vi "Lab Panel V4.91.vi"() -> ()   [LabVIEW 2013] (continued)
              n208 = local read "SIG LAB02-1"() -> (w244:T2)
              n209 = local read "SIG LAB02-2"() -> (w243:T2)
              n210 = local read "TEMP LA02"() -> (w248:T9)
              n211 = Bundle By Name(cluster=w248, "TL-1"=w240, "TN-1"=w239, "TL-2"=w238, "TN-2"=w237, "TL -1COUNT"=w245, "TN-1 COUNT"=w245, "TL-2 COUNT"=w245, "TN-2 COUNT"=w245) -> (w246:T9)
              n212 = Bundle(cluster=w243, "Tmp Live"=w238, "Tmp Neut"=w237) -> (w241:T2)  [unwired: 3 in]
              n213 = Bundle(cluster=w244, "Tmp Live"=w240, "Tmp Neut"=w239) -> (w242:T2)  [unwired: 3 in]
              n214 = local write "TEMP LA02"(w246) -> ()
              n215 = local write "SIG LAB02-1"(w242) -> ()
              n216 = local write "SIG LAB02-2"(w241) -> ()
            }
            frame #4 {
              w257 = 0
              n217 = local read "LAB03 TEMP"() -> (w259:T12)
              n218 = Unbundle By Name(w259) -> ("T1 Live"=w252:dbl, "T1 Neut"=w251:dbl, "T2 Live"=w250:dbl, "T2 Neut"=w249:dbl)  [unwired: 2 out]
              n219 = local read "SIG LAB03-1"() -> (w256:T2)
              n220 = local read "SIG LAB03-2"() -> (w255:T2)
              n221 = local read "TEMP LA03"() -> (w260:T9)
              n222 = Bundle By Name(cluster=w260, "TL-1"=w252, "TN-1"=w251, "TL-2"=w250, "TN-2"=w249, "TL -1COUNT"=w257, "TN-1 COUNT"=w257, "TL-2 COUNT"=w257, "TN-2 COUNT"=w257) -> (w258:T9)
              n223 = Bundle(cluster=w255, "Tmp Live"=w250, "Tmp Neut"=w249) -> (w253:T2)  [unwired: 3 in]
              n224 = Bundle(cluster=w256, "Tmp Live"=w252, "Tmp Neut"=w251) -> (w254:T2)  [unwired: 3 in]
              n225 = local write "TEMP LA03"(w258) -> ()
              n226 = local write "SIG LAB03-2"(w253) -> ()
              n227 = local write "SIG LAB03-1"(w254) -> ()
            }
            frame #5 {
              w269 = 0
              n228 = local read "LAB04 TEMP"() -> (w271:T12)
              n229 = Unbundle By Name(w271) -> ("T1 Live"=w264:dbl, "T1 Neut"=w263:dbl, "T2 Live"=w262:dbl, "T2 Neut"=w261:dbl)  [unwired: 2 out]
              n230 = local read "SIG LAB04-2"() -> (w267:T2)
              n231 = local read "SIG LAB04-1"() -> (w268:T2)
              n232 = local read "TEMP LA04"() -> (w272:T9)
              n233 = Bundle By Name(cluster=w272, "TL-1"=w264, "TN-1"=w263, "TL-2"=w262, "TN-2"=w261, "TL -1COUNT"=w269, "TN-1 COUNT"=w269, "TL-2 COUNT"=w269, "TN-2 COUNT"=w269) -> (w270:T9)
              n234 = Bundle(cluster=w267, "Tmp Live"=w262, "Tmp Neut"=w261) -> (w265:T2)  [unwired: 3 in]
              n235 = Bundle(cluster=w268, "Tmp Live"=w264, "Tmp Neut"=w263) -> (w266:T2)  [unwired: 3 in]
              n236 = local write "SIG LAB04-2"(w265) -> ()
              n237 = local write "TEMP LA04"(w270) -> ()
              n238 = local write "SIG LAB04-1"(w266) -> ()
            }
            frame #6 {
              w281 = 0
              n239 = local read "LAB05 TEMP"() -> (w283:T12)
              n240 = Unbundle By Name(w283) -> ("T1 Live"=w276:dbl, "T1 Neut"=w275:dbl, "T2 Live"=w274:dbl, "T2 Neut"=w273:dbl)  [unwired: 2 out]
              n241 = local read "SIG LAB05-2"() -> (w279:T2)
              n242 = local read "SIG LAB05-1"() -> (w280:T2)
              n243 = local read "TEMP LA05"() -> (w284:T9)
              n244 = Bundle By Name(cluster=w284, "TL-1"=w276, "TN-1"=w275, "TL-2"=w274, "TN-2"=w273, "TL -1COUNT"=w281, "TN-1 COUNT"=w281, "TL-2 COUNT"=w281, "TN-2 COUNT"=w281) -> (w282:T9)
              n245 = Bundle(cluster=w279, "Tmp Live"=w274, "Tmp Neut"=w273) -> (w277:T2)  [unwired: 3 in]
              n246 = Bundle(cluster=w280, "Tmp Live"=w276, "Tmp Neut"=w275) -> (w278:T2)  [unwired: 3 in]
              n247 = local write "SIG LAB05-2"(w277) -> ()
              n248 = local write "SIG LAB05-1"(w278) -> ()
              n249 = local write "TEMP LA05"(w282) -> ()
            }
          }
        }
        frame #8 {
          # "enable front panel, all settings done"
          n250 = property on="Tab Control 2" class="TabCtl (strict)"("DisabledEnum"=T16."Enabled" ("Disabled")) -> ()  [unwired: 2 in, 2 out]
          n251 = property on="Tab Control 2" class="TabCtl (strict)"("Value"=0) -> ()  [unwired: 2 in, 2 out]
        }
        frame #9 {
          n252 = property on="Tab Control 2" class="TabCtl (strict)"("Value"=0) -> ()  [unwired: 2 in, 2 out]
        }
      }
    }
    frame #2 {
      n253 = node-c288("loop  delay(mS)") -> (w290:T17)  [unwired: 3 in]
      n254 = timed-loop {
        timing: w290 -> [_]
        timing-out: [_] -> w289
        i -> [w312]
        stop <- "stop" stop-if-true
        n255 = node-c288() -> ()  [unwired: 1 in, 1 out]
        n256 = global write "Global display 1.vi" "stop disp"("stop") -> ()
        n257 = local read "SELECT LAB05-2"() -> (w292:T3)
        n258 = local read "SELECT LAB05-1"() -> (w293:T3)
        n259 = local read "SELECT LAB04-2"() -> (w294:T3)
        n260 = local read "SELECT LAB03-1"() -> (w297:T3)
        n261 = local read "SELECT LAB02-2"() -> (w298:T3)
        n262 = local read "SELECT LAB01-1"() -> (w301:T3)
        n263 = local read "SELECT LAB03-2"() -> (w296:T3)
        n264 = local read "SELECT LAB01-2"() -> (w300:T3)
        n265 = local read "SELECT LAB04-1"() -> (w295:T3)
        n266 = local read "SELECT LAB02-1"() -> (w299:T3)
        n267 = local read "run lab03-2"() -> (w306:bool)
        n268 = local read "run lab04-1"() -> (w305:bool)
        n269 = local read "run lab05-1"() -> (w303:bool)
        n270 = local read "run lab04-2"() -> (w304:bool)
        n271 = local read "run lab05-2"() -> (w302:bool)
        n272 = local read "run lab03-1"() -> (w307:bool)
        n273 = local read "run lab02-2"() -> (w308:bool)
        n274 = local read "run lab02-1"() -> (w309:bool)
        n275 = local read "run lab01-1"() -> (w311:bool)
        n276 = local read "run lab01-2"() -> (w310:bool)
        n277 = stacked-sequence {
          seq-local: [_ w377 _ _ _ _ _ _ _ _ _ _ _ _ _ _ _ _ _ _ _ _ _] -> [_ _ _ _ _ w2478 _ _ _ _ _ _ _ _ _ _ _ _ _ _ _ _ _]
          seq-local: [_ w376 _ _ _ _ _ _ _ _ _ _ _ _ _ _ _ _ _ _ _ _ _] -> [_ _ _ _ _ w2477 _ _ _ _ _ _ _ _ _ _ _ _ _ _ _ _ _]
          seq-local: [_ w363 _ _ _ _ _ _ _ _ _ _ _ _ _ _ _ _ _ _ _ _ _] -> [_ _ _ _ _ w2476 _ _ _ _ _ _ _ _ _ _ _ _ _ _ _ _ _]
          seq-local: [_ w362 _ _ _ _ _ _ _ _ _ _ _ _ _ _ _ _ _ _ _ _ _] -> [_ _ _ _ _ w2475 _ _ _ _ _ _ _ _ _ _ _ _ _ _ _ _ _]
          seq-local: [_ w361 _ _ _ _ _ _ _ _ _ _ _ _ _ _ _ _ _ _ _ _ _] -> [_ _ _ _ _ w2474 _ _ _ _ _ _ _ _ _ _ _ _ _ _ _ _ _]
          seq-local: [_ w360 _ _ _ _ _ _ _ _ _ _ _ _ _ _ _ _ _ _ _ _ _] -> [_ _ _ _ _ w2473 _ _ _ _ _ _ _ _ _ _ _ _ _ _ _ _ _]
          seq-local: [_ w359 _ _ _ _ _ _ _ _ _ _ _ _ _ _ _ _ _ _ _ _ _] -> [_ _ _ _ _ w2472 _ _ _ _ _ _ _ _ _ _ _ _ _ _ _ _ _]
          seq-local: [_ w358 _ _ _ _ _ _ _ _ _ _ _ _ _ _ _ _ _ _ _ _ _] -> [_ _ _ _ _ w2471 _ _ _ _ _ _ _ _ _ _ _ _ _ _ _ _ _]
          seq-local: [_ w357 _ _ _ _ _ _ _ _ _ _ _ _ _ _ _ _ _ _ _ _ _] -> [_ _ _ _ _ w2470 _ _ _ _ _ _ _ _ _ _ _ _ _ _ _ _ _]
          seq-local: [_ w356 _ _ _ _ _ _ _ _ _ _ _ _ _ _ _ _ _ _ _ _ _] -> [_ _ _ _ _ w2469 _ _ _ _ _ _ _ _ _ _ _ _ _ _ _ _ _]
          tunnel: w311 -> [_ _ w393 w641 w2068 w2498 w2813 w3300 _ _ _ _ w3725 _ w4682 _ _ w4969 w5272 w5454 _ _ _]
          tunnel: w310 -> [_ _ w392 w639 w2067 w2497 w2814 w3299 _ _ _ _ w3724 _ w4680 _ _ w4968 w5271 w5452 _ _ _]
          tunnel: w309 -> [_ _ w391 w637 w2066 w2496 w2812 w3298 _ _ _ _ w3723 _ w4678 _ _ w4967 w5270 w5451 _ _ _]
          tunnel: w308 -> [_ _ w390 w635 w2065 w2495 w2811 w3297 _ _ _ _ w3722 _ w4676 _ _ w4966 w5269 w5450 _ _ _]
          tunnel: w307 -> [_ _ w389 w633 w2064 w2494 w2810 w3296 _ _ _ _ w3721 _ w4674 _ _ w4965 w5268 w5449 _ _ _]
          tunnel: w306 -> [_ _ w388 w631 w2063 w2493 w2809 w3295 _ _ _ _ w3720 _ w4672 _ _ w4964 w5267 w5448 _ _ _]
          tunnel: w305 -> [_ _ w387 w629 w2062 w2492 w2808 w3294 _ _ _ _ w3719 _ w4670 _ _ w4963 w5266 w5447 _ _ _]
          tunnel: w304 -> [_ _ w386 w627 w2061 w2491 w2807 w3293 _ _ _ _ w3718 _ w4668 _ _ w4962 w5265 w5446 _ _ _]
          tunnel: w303 -> [_ _ w385 w625 w2060 w2490 w2806 w3292 _ _ _ _ w3717 _ w4666 _ _ w4961 w5264 w5445 _ _ _]
          tunnel: w302 -> [_ _ w384 w623 w2059 w2489 w2805 w3291 _ _ _ _ w3716 _ w4664 _ _ w4960 w5263 w5444 _ _ _]
          tunnel: w301 -> [_ _ _ w640 w2058 w2488 _ _ _ _ _ _ _ _ w4684 _ _ _ _ _ w5792 _ _]
          tunnel: w300 -> [_ _ _ w638 w2057 w2487 _ _ _ _ _ _ _ _ w4679 _ _ _ _ _ w5791 _ _]
          tunnel: w299 -> [_ _ _ w636 w2056 w2486 _ _ _ _ _ _ _ _ w4677 _ _ _ _ _ w5790 _ _]
          tunnel: w298 -> [_ _ _ w634 w2055 w2485 _ _ _ _ _ _ _ _ w4675 _ _ _ _ _ w5789 _ _]
          tunnel: w297 -> [_ _ _ w632 w2054 w2484 _ _ _ _ _ _ _ _ w4673 _ _ _ _ _ w5788 _ _]
          tunnel: w296 -> [_ _ _ w630 w2053 w2483 _ _ _ _ _ _ _ _ w4671 _ _ _ _ _ w5787 _ _]
          tunnel: w295 -> [_ _ _ w628 w2052 w2482 _ _ _ _ _ _ _ _ w4669 _ _ _ _ _ w5786 _ _]
          tunnel: w294 -> [_ _ _ w626 w2051 w2481 _ _ _ _ _ _ _ _ w4667 _ _ _ _ _ w5785 _ _]
          tunnel: w293 -> [_ _ _ w624 w2050 w2480 _ _ _ _ _ _ _ _ w4665 _ _ _ _ _ w5784 _ _]
          tunnel: w292 -> [_ _ _ w622 w2049 w2479 _ _ _ _ _ _ _ _ w4663 _ _ _ _ _ w5783 _ _]
          frame #0 {
            w319 = FALSE
            w324 = 0.5
            # "set up cycle control"
            n278 = local read "jig cycle"() -> (w323:dbl)
            n279 = local read "Amps Fail level"() -> (w317:dbl)
            n280 = Divide(x="JIG ON TIME (S)", y=w324) -> (x/y=→"on loops":dbl)
            n281 = Divide(x="JIG OFF TIME (S)", y=w324) -> (x/y=→"off loops":dbl)
            n282 = global write "Global display 3.vi" "Amps Fail"(w317) -> ()
            n283 = Increment(x=w323) -> (x+1=w322:dbl)
            n284 = local write "TEMP"(w319) -> ()
            n285 = local write "AI"(w319) -> ()
            n286 = local read "Network Directory"() -> (w316:path)
            n287 = local write "jig cycle"(w322) -> ()
            n288 = call "sub vi - check network dir v2.vi"("PATH"=w316) -> ("error"=w315:bool)  [unwired: 10 in]
            n289 = local write "network error"(w315) -> ()
            n290 = global write "Global display 3.vi" "network drive"(w315) -> ()
            n291 = event shown="[1] \"ADMIN\": Value Change" {
              selector: _ -> [_ _]
              dyn-events: _ -> [_ _]
              timeout: 10 -> [_ _]
              event Timeout {
                n292 = event-data() -> ()  [unwired: 1 in, 3 out]
              }
              event "ADMIN": Value Change {
                n293 = event-data() -> ()  [unwired: 1 in, 6 out]
                n294 = stacked-sequence {
                  seq-local: [_ w328 _] -> [_ _ w329]
                  frame #0 {
                    n295 = global write "Global 1.vi" "password"("9949") -> ()
                  }
                  frame #1 {
                    n296 = call "sub vi - password 1.vi"() -> ("RESULT"=w328:bool)  [unwired: 11 in]
                  }
                  frame #2 {
                    w331 = FALSE
                    n297 = property on="Tab Control 2" class="TabCtl (strict)"() -> ("Pages"=w335:refnum<vi>[])  [unwired: 2 in, 2 out]
                    n298 = Select(t=TRUE, s=w329, f=w331) -> (s? t:f=w330:bool)
                    n299 = Index Array(array=w335, index=8) -> (element=w333:refnum<vi>)
                    n300 = property class="Page"(reference=w333, "PageVis"=w330) -> ()  [unwired: 1 in, 2 out]
                    n301 = local write "ADMIN"(w331) -> ()
                  }
                }
              }
            }
          }
          frame #1 {
            w373 = 60.0
            # "convert temperature rise minutes to cycles"
            n302 = local read "SET LAB05-2"() -> (w337:T5)
            n303 = local read "SET LAB05-1"() -> (w339:T5)
            n304 = local read "SET LAB04-2"() -> (w341:T5)
            n305 = local read "SET LAB01-1"() -> (w355:T5)
            n306 = local read "SET LAB01-2"() -> (w353:T5)
            n307 = local read "SET LAB02-2"() -> (w349:T5)
            n308 = local read "SET LAB04-1"() -> (w343:T5)
            n309 = local read "SET LAB03-1"() -> (w347:T5)
            n310 = local read "SET LAB03-2"() -> (w345:T5)
            n311 = local read "SET LAB02-1"() -> (w351:T5)
            n312 = local read "JIG OFF TIME (S)"() -> (w378:dbl)
            n313 = local read "JIG ON TIME (S)"() -> (w379:dbl)
            n314 = Unbundle(w337) -> ("T-RISE mins"=w336:dbl)  [unwired: 4 out]
            n315 = Unbundle(w339) -> ("T-RISE mins"=w338:dbl)  [unwired: 4 out]
            n316 = Unbundle(w355) -> ("T-RISE mins"=w354:dbl)  [unwired: 4 out]
            n317 = Unbundle(w341) -> ("T-RISE mins"=w340:dbl)  [unwired: 4 out]
            n318 = Unbundle(w353) -> ("T-RISE mins"=w352:dbl)  [unwired: 4 out]
            n319 = Unbundle(w351) -> ("T-RISE mins"=w350:dbl)  [unwired: 4 out]
            n320 = Unbundle(w343) -> ("T-RISE mins"=w342:dbl)  [unwired: 4 out]
            n321 = Unbundle(w349) -> ("T-RISE mins"=w348:dbl)  [unwired: 4 out]
            n322 = Unbundle(w345) -> ("T-RISE mins"=w344:dbl)  [unwired: 4 out]
            n323 = Unbundle(w347) -> ("T-RISE mins"=w346:dbl)  [unwired: 4 out]
            n324 = Add(x=w379, y=w378) -> (x+y=w372:dbl)
            n325 = Multiply(x=w373, y=w344) -> (x*y=w368:dbl)
            n326 = Multiply(x=w373, y=w342) -> (x*y=w367:dbl)
            n327 = Multiply(x=w373, y=w340) -> (x*y=w366:dbl)
            n328 = Multiply(x=w373, y=w338) -> (x*y=w365:dbl)
            n329 = Multiply(x=w373, y=w336) -> (x*y=w364:dbl)
            n330 = Multiply(x=w373, y=w352) -> (x*y=w374:dbl)
            n331 = Multiply(x=w373, y=w346) -> (x*y=w369:dbl)
            n332 = Multiply(x=w373, y=w354) -> (x*y=w375:dbl)
            n333 = Multiply(x=w373, y=w350) -> (x*y=w371:dbl)
            n334 = Multiply(x=w373, y=w348) -> (x*y=w370:dbl)
            n335 = Divide(x=w365, y=w372) -> (x/y=w357:dbl)
            n336 = Divide(x=w366, y=w372) -> (x/y=w358:dbl)
            n337 = Divide(x=w367, y=w372) -> (x/y=w359:dbl)
            n338 = Divide(x=w364, y=w372) -> (x/y=w356:dbl)
            n339 = Divide(x=w369, y=w372) -> (x/y=w361:dbl)
            n340 = Divide(x=w375, y=w372) -> (x/y=w377:dbl)
            n341 = Divide(x=w374, y=w372) -> (x/y=w376:dbl)
            n342 = Divide(x=w371, y=w372) -> (x/y=w363:dbl)
            n343 = Divide(x=w370, y=w372) -> (x/y=w362:dbl)
            n344 = Divide(x=w368, y=w372) -> (x/y=w360:dbl)
          }
          frame #2 {
            # "control cycle loops"
            n345 = local read "JIG OFF TIME (S)"() -> (w382:dbl)
            n346 = local read "JIG ON TIME (S)"() -> (w381:dbl)
            n347 = local read "jig cycle"() -> (w395:dbl)
            n348 = local read "on loops"() -> (w397:dbl)
            n349 = local read "off loops"() -> (w396:dbl)
            n350 = Add(x=w382, y=w381) -> (x+y=w380:dbl)
            n351 = Add(x=w397, y=w396) -> (x+y=w383:dbl)
            n352 = Greater Or Equal?(x=w395, y=w383) -> (x >= y?=w394:bool)
            n353 = case shown="True" w394 {
              tunnel: w393 -> [_ w431]
              tunnel: w392 -> [_ w430]
              tunnel: w391 -> [_ w429]
              tunnel: w390 -> [_ w428]
              tunnel: w389 -> [_ w427]
              tunnel: w388 -> [_ w426]
              tunnel: w387 -> [_ w425]
              tunnel: w386 -> [_ w424]
              tunnel: w385 -> [_ w423]
              tunnel: w384 -> [_ w422]
              tunnel: w380 -> [_ w421]
              frame False {
              }
              frame True {
                # "increment cycle value and convert cycles to minutes for temp rise"
                n354 = stacked-sequence {
                  frame #0 {
                    n355 = local read "Panel #"() -> (w434:dbl)
                    n356 = Increment(x=w434) -> (x+1=w433:dbl)
                    n357 = local write "Panel #"(w433) -> ()
                  }
                  frame #1 {
                    n358 = local read "Panel #"() -> (w435:dbl)
                    n359 = Greater?(x=w435, y=5) -> (0:w437:bool)
                    n360 = case shown="True" w437 {
                      frame False {
                      }
                      frame True {
                        n361 = local write "Panel #"(1) -> ()
                      }
                    }
                  }
                }
                n362 = local read "JIG RELAY CYCLES"() -> (w420:T8)
                n363 = local read "Panel #"() -> (→"Tmp Upd":dbl)
                n364 = Unbundle By Name(w420) -> ("LAB01-1"=w418:dbl, "LAB01-2"=w416:dbl, "LAB02-1"=w414:dbl, "LAB02-2"=w412:dbl, "LAB03-1"=w410:dbl, "LAB03-2"=w408:dbl, "LAB04-1"=w406:dbl, "LAB04-2"=w404:dbl, "LAB05-1"=w402:dbl, "LAB05-2"=w400:dbl)
                n365 = stacked-sequence {
                  tunnel: w431 -> [w449 _ _ _ _ _ _ _ _ _]
                  tunnel: w430 -> [_ w466 _ _ _ _ _ _ _ _]
                  tunnel: w429 -> [_ _ w483 _ _ _ _ _ _ _]
                  tunnel: w428 -> [_ _ _ w500 _ _ _ _ _ _]
                  tunnel: w427 -> [_ _ _ _ w517 _ _ _ _ _]
                  tunnel: w426 -> [_ _ _ _ _ w534 _ _ _ _]
                  tunnel: w425 -> [_ _ _ _ _ _ w551 _ _ _]
                  tunnel: w424 -> [_ _ _ _ _ _ _ w568 _ _]
                  tunnel: w423 -> [_ _ _ _ _ _ _ _ w585 _]
                  tunnel: w422 -> [_ _ _ _ _ _ _ _ _ w602]
                  tunnel: w421 -> [w446 w463 w480 w497 w514 w531 w548 w565 w582 w599]
                  tunnel: w418 -> [w440 _ _ _ _ _ _ _ _ _]
                  tunnel: [w439 _ _ _ _ _ _ _ _ _] -> w417
                  tunnel: w416 -> [_ w457 _ _ _ _ _ _ _ _]
                  tunnel: [_ w456 _ _ _ _ _ _ _ _] -> w415
                  tunnel: w414 -> [_ _ w474 _ _ _ _ _ _ _]
                  tunnel: [_ _ w473 _ _ _ _ _ _ _] -> w413
                  tunnel: w412 -> [_ _ _ w491 _ _ _ _ _ _]
                  tunnel: [_ _ _ w490 _ _ _ _ _ _] -> w411
                  tunnel: w410 -> [_ _ _ _ w508 _ _ _ _ _]
                  tunnel: [_ _ _ _ w507 _ _ _ _ _] -> w409
                  tunnel: w408 -> [_ _ _ _ _ w525 _ _ _ _]
                  tunnel: [_ _ _ _ _ w524 _ _ _ _] -> w407
                  tunnel: w406 -> [_ _ _ _ _ _ w542 _ _ _]
                  tunnel: [_ _ _ _ _ _ w541 _ _ _] -> w405
                  tunnel: w404 -> [_ _ _ _ _ _ _ w559 _ _]
                  tunnel: [_ _ _ _ _ _ _ w558 _ _] -> w403
                  tunnel: w402 -> [_ _ _ _ _ _ _ _ w576 _]
                  tunnel: [_ _ _ _ _ _ _ _ w575 _] -> w401
                  tunnel: w400 -> [_ _ _ _ _ _ _ _ _ w593]
                  tunnel: [_ _ _ _ _ _ _ _ _ w592] -> w399
                  frame #0 {
                    n366 = local read "DISP LAB01-1"() -> (w444:T4)
                    n367 = Unbundle(w444) -> ("CYCLE"=w445:dbl)  [unwired: 2 out]
                    n368 = case shown="True" w449 {
                      tunnel: w445 -> [w451 w455]
                      tunnel: [w451 w454] -> w443
                      tunnel: w440 -> [w450 w453]
                      tunnel: [w450 w452] -> w439
                      frame False {
                      }
                      frame True {
                        n369 = Increment(x=w453) -> (x+1=w452:dbl)
                        n370 = Increment(x=w455) -> (x+1=w454:dbl)
                      }
                    }
                    n371 = Multiply(x=w443, y=w446) -> (x*y=w447:dbl)
                    n372 = Divide(x=w447, y=60.0) -> (x/y=w442:dbl)
                    n373 = Bundle(cluster=w444, "CYCLE"=w443, "MINS"=w442) -> (w441:T4)  [unwired: 1 in]
                    n374 = local write "DISP LAB01-1"(w441) -> ()
                  }
                  frame #1 {
                    n375 = local read "DISP LAB01-2"() -> (w461:T4)
                    n376 = Unbundle(w461) -> ("CYCLE"=w462:dbl)  [unwired: 2 out]
                    n377 = case shown="True" w466 {
                      tunnel: w462 -> [w468 w472]
                      tunnel: [w468 w471] -> w459
                      tunnel: w457 -> [w467 w470]
                      tunnel: [w467 w469] -> w456
                      frame False {
                      }
                      frame True {
                        n378 = Increment(x=w470) -> (x+1=w469:dbl)
                        n379 = Increment(x=w472) -> (x+1=w471:dbl)
                      }
                    }
                    n380 = Multiply(x=w459, y=w463) -> (x*y=w464:dbl)
                    n381 = Divide(x=w464, y=60.0) -> (x/y=w458:dbl)
                    n382 = Bundle(cluster=w461, "CYCLE"=w459, "MINS"=w458) -> (w460:T4)  [unwired: 1 in]
                    n383 = local write "DISP LAB01-2"(w460) -> ()
                  }
                  frame #2 {
                    n384 = local read "DISP LAB02-1"() -> (w478:T4)
                    n385 = Unbundle(w478) -> ("CYCLE"=w479:dbl)  [unwired: 2 out]
                    n386 = case shown="True" w483 {
                      tunnel: [w485 w489] -> w476
                      tunnel: w479 -> [w485 w488]
                      tunnel: w474 -> [w484 w487]
                      tunnel: [w484 w486] -> w473
                      frame False {
                      }
                      frame True {
                        n387 = Increment(x=w487) -> (x+1=w486:dbl)
                        n388 = Increment(x=w488) -> (x+1=w489:dbl)
                      }
                    }
                    n389 = Multiply(x=w476, y=w480) -> (x*y=w481:dbl)
                    n390 = Divide(x=w481, y=60.0) -> (x/y=w475:dbl)
                    n391 = Bundle(cluster=w478, "CYCLE"=w476, "MINS"=w475) -> (w477:T4)  [unwired: 1 in]
                    n392 = local write "DISP LAB02-1"(w477) -> ()
                  }
                  frame #3 {
                    n393 = local read "DISP LAB02-2"() -> (w495:T4)
                    n394 = Unbundle(w495) -> ("CYCLE"=w496:dbl)  [unwired: 2 out]
                    n395 = case shown="True" w500 {
                      tunnel: [w502 w506] -> w494
                      tunnel: w496 -> [w502 w505]
                      tunnel: w491 -> [w501 w504]
                      tunnel: [w501 w503] -> w490
                      frame False {
                      }
                      frame True {
                        n396 = Increment(x=w504) -> (x+1=w503:dbl)
                        n397 = Increment(x=w505) -> (x+1=w506:dbl)
                      }
                    }
                    n398 = Multiply(x=w494, y=w497) -> (x*y=w498:dbl)
                    n399 = Divide(x=w498, y=60.0) -> (x/y=w493:dbl)
                    n400 = Bundle(cluster=w495, "CYCLE"=w494, "MINS"=w493) -> (w492:T4)  [unwired: 1 in]
                    n401 = local write "DISP LAB02-2"(w492) -> ()
                  }
                  frame #4 {
                    n402 = local read "DISP LAB03-1"() -> (w512:T4)
                    n403 = Unbundle(w512) -> ("CYCLE"=w513:dbl)  [unwired: 2 out]
                    n404 = case shown="True" w517 {
                      tunnel: [w519 w523] -> w509
                      tunnel: w513 -> [w519 w522]
                      tunnel: w508 -> [w518 w521]
                      tunnel: [w518 w520] -> w507
                      frame False {
                      }
                      frame True {
                        n405 = Increment(x=w521) -> (x+1=w520:dbl)
                        n406 = Increment(x=w522) -> (x+1=w523:dbl)
                      }
                    }
                    n407 = Multiply(x=w509, y=w514) -> (x*y=w515:dbl)
                    n408 = Divide(x=w515, y=60.0) -> (x/y=w510:dbl)
                    n409 = Bundle(cluster=w512, "CYCLE"=w509, "MINS"=w510) -> (w511:T4)  [unwired: 1 in]
                    n410 = local write "DISP LAB03-1"(w511) -> ()
                  }
                  frame #5 {
                    n411 = local read "DISP LAB03-2"() -> (w529:T4)
                    n412 = Unbundle(w529) -> ("CYCLE"=w530:dbl)  [unwired: 2 out]
                    n413 = case shown="True" w534 {
                      tunnel: [w536 w540] -> w528
                      tunnel: w530 -> [w536 w539]
                      tunnel: w525 -> [w535 w538]
                      tunnel: [w535 w537] -> w524
                      frame False {
                      }
                      frame True {
                        n414 = Increment(x=w538) -> (x+1=w537:dbl)
                        n415 = Increment(x=w539) -> (x+1=w540:dbl)
                      }
                    }
                    n416 = Multiply(x=w528, y=w531) -> (x*y=w532:dbl)
                    n417 = Divide(x=w532, y=60.0) -> (x/y=w527:dbl)
                    n418 = Bundle(cluster=w529, "CYCLE"=w528, "MINS"=w527) -> (w526:T4)  [unwired: 1 in]
                    n419 = local write "DISP LAB03-2"(w526) -> ()
                  }
                  frame #6 {
                    n420 = local read "DISP LAB04-1"() -> (w546:T4)
                    n421 = Unbundle(w546) -> ("CYCLE"=w547:dbl)  [unwired: 2 out]
                    n422 = case shown="True" w551 {
                      tunnel: [w553 w557] -> w544
                      tunnel: w547 -> [w553 w556]
                      tunnel: w542 -> [w552 w555]
                      tunnel: [w552 w554] -> w541
                      frame False {
                      }
                      frame True {
                        n423 = Increment(x=w555) -> (x+1=w554:dbl)
                        n424 = Increment(x=w556) -> (x+1=w557:dbl)
                      }
                    }
                    n425 = Multiply(x=w544, y=w548) -> (x*y=w549:dbl)
                    n426 = Divide(x=w549, y=60.0) -> (x/y=w543:dbl)
                    n427 = Bundle(cluster=w546, "CYCLE"=w544, "MINS"=w543) -> (w545:T4)  [unwired: 1 in]
                    n428 = local write "DISP LAB04-1"(w545) -> ()
                  }
                  frame #7 {
                    n429 = local read "DISP LAB04-2"() -> (w563:T4)
                    n430 = Unbundle(w563) -> ("CYCLE"=w564:dbl)  [unwired: 2 out]
                    n431 = case shown="True" w568 {
                      tunnel: [w570 w574] -> w561
                      tunnel: w564 -> [w570 w573]
                      tunnel: w559 -> [w569 w572]
                      tunnel: [w569 w571] -> w558
                      frame False {
                      }
                      frame True {
                        n432 = Increment(x=w572) -> (x+1=w571:dbl)
                        n433 = Increment(x=w573) -> (x+1=w574:dbl)
                      }
                    }
                    n434 = Multiply(x=w561, y=w565) -> (x*y=w567:dbl)
                    n435 = Divide(x=w567, y=60.0) -> (x/y=w560:dbl)
                    n436 = Bundle(cluster=w563, "CYCLE"=w561, "MINS"=w560) -> (w562:T4)  [unwired: 1 in]
                    n437 = local write "DISP LAB04-2"(w562) -> ()
                  }
                  frame #8 {
                    n438 = local read "DISP LAB05-1"() -> (w580:T4)
                    n439 = Unbundle(w580) -> ("CYCLE"=w581:dbl)  [unwired: 2 out]
                    n440 = case shown="True" w585 {
                      tunnel: [w587 w591] -> w578
                      tunnel: w581 -> [w587 w590]
                      tunnel: w576 -> [w586 w589]
                      tunnel: [w586 w588] -> w575
                      frame False {
                      }
                      frame True {
                        n441 = Increment(x=w589) -> (x+1=w588:dbl)
                        n442 = Increment(x=w590) -> (x+1=w591:dbl)
                      }
                    }
                    n443 = Multiply(x=w578, y=w582) -> (x*y=w583:dbl)
                    n444 = Divide(x=w583, y=60.0) -> (x/y=w577:dbl)
                    n445 = Bundle(cluster=w580, "CYCLE"=w578, "MINS"=w577) -> (w579:T4)  [unwired: 1 in]
                    n446 = local write "DISP LAB05-1"(w579) -> ()
                  }
                  frame #9 {
                    n447 = local read "DISP LAB05-2"() -> (w598:T4)
                    n448 = Unbundle(w598) -> ("CYCLE"=w597:dbl)  [unwired: 2 out]
                    n449 = case shown="True" w602 {
                      tunnel: [w604 w608] -> w596
                      tunnel: w597 -> [w604 w607]
                      tunnel: w593 -> [w603 w606]
                      tunnel: [w603 w605] -> w592
                      frame False {
                      }
                      frame True {
                        n450 = Increment(x=w606) -> (x+1=w605:dbl)
                        n451 = Increment(x=w607) -> (x+1=w608:dbl)
                      }
                    }
                    n452 = Multiply(x=w596, y=w599) -> (x*y=w600:dbl)
                    n453 = Divide(x=w600, y=60.0) -> (x/y=w595:dbl)
                    n454 = Bundle(cluster=w598, "CYCLE"=w596, "MINS"=w595) -> (w594:T4)  [unwired: 1 in]
                    n455 = local write "DISP LAB05-2"(w594) -> ()
                  }
                }
                n456 = local write "jig cycle"(0) -> ()
                n457 = Bundle By Name(cluster=w420, "LAB01-1"=w417, "LAB01-2"=w415, "LAB02-1"=w413, "LAB02-2"=w411, "LAB03-1"=w409, "LAB03-2"=w407, "LAB04-1"=w405, "LAB04-2"=w403, "LAB05-1"=w401, "LAB05-2"=w399) -> (w419:T8)
                n458 = local write "JIG RELAY CYCLES"(w419) -> ()
              }
            }
          }
          frame #3 {
            # "START & STOP test RUN switch change, start test if true and stop test if false"
            n459 = Get Date/Time In Seconds() -> (seconds since 1Jan1904=w620:timestamp)
            n460 = local read "C drive data root dir"() -> (w613:path)
            n461 = Format Date/Time String(time format string (%c)="%b\\%a%d", seconds (now)=w620) -> (date/time string=w644:string)  [unwired: 1 in]
            n462 = Format Date/Time String(time format string (%c)="%H%M", seconds (now)=w620) -> (date/time string=w642:string)  [unwired: 1 in]
            n463 = Format Date/Time String(time format string (%c)="LabPanel%Y", seconds (now)=w620) -> (date/time string=w619:string)  [unwired: 1 in]
            n464 = Path To String(path=w613) -> (string=w616:string)
            n465 = global write "Global 1.vi" "C drive root path"(w613) -> ()
            n466 = local read "Ref deg C"() -> (w609:dbl)
            n467 = Concatenate Strings(w616, "\\") -> (w614:string)
            n468 = event shown="[1] \"RUN LAB01-1\": Value Change" {
              selector: _ -> [_ _ _ _ _ _ _ _ _ _ _]
              dyn-events: _ -> [_ _ _ _ _ _ _ _ _ _ _]
              timeout: 10 -> [_ _ _ _ _ _ _ _ _ _ _]
              tunnel: w614 -> [_ w657 w797 w938 w1078 w1218 w1358 w1498 w1638 w1778 w1919]
              tunnel: w644 -> [_ w656 w796 w937 w1077 w1217 w1357 w1497 w1637 w1777 w1918]
              tunnel: w642 -> [_ w654 w795 w936 w1076 w1216 w1356 w1496 w1636 w1776 w1917]
              tunnel: w640 -> [_ w655 _ _ _ _ _ _ _ _ _]
              tunnel: w641 -> [_ _ _ _ _ _ _ _ _ _ _]
              tunnel: w639 -> [_ _ _ _ _ _ _ _ _ _ _]
              tunnel: w638 -> [_ _ w794 _ _ _ _ _ _ _ _]
              tunnel: w637 -> [_ _ _ _ _ _ _ _ _ _ _]
              tunnel: w636 -> [_ _ _ w935 _ _ _ _ _ _ _]
              tunnel: w635 -> [_ _ _ _ _ _ _ _ _ _ _]
              tunnel: w634 -> [_ _ _ _ w1075 _ _ _ _ _ _]
              tunnel: w633 -> [_ _ _ _ _ _ _ _ _ _ _]
              tunnel: w632 -> [_ _ _ _ _ w1215 _ _ _ _ _]
              tunnel: w631 -> [_ _ _ _ _ _ _ _ _ _ _]
              tunnel: w630 -> [_ _ _ _ _ _ w1355 _ _ _ _]
              tunnel: w629 -> [_ _ _ _ _ _ _ _ _ _ _]
              tunnel: w628 -> [_ _ _ _ _ _ _ w1495 _ _ _]
              tunnel: w627 -> [_ _ _ _ _ _ _ _ _ _ _]
              tunnel: w626 -> [_ _ _ _ _ _ _ _ w1635 _ _]
              tunnel: w625 -> [_ _ _ _ _ _ _ _ _ _ _]
              tunnel: w624 -> [_ _ _ _ _ _ _ _ _ w1775 _]
              tunnel: w623 -> [_ _ _ _ _ _ _ _ _ _ _]
              tunnel: w622 -> [_ _ _ _ _ _ _ _ _ _ w1916]
              tunnel: w619 -> [_ w653 w793 w934 w1074 w1214 w1354 w1494 w1634 w1774 w1915]
              tunnel: [_ w652 w792 w933 w1073 w1213 w1353 w1493 w1633 w1773 w1914] -> w617
              tunnel: "RESET CYCLES TO ZERO?" -> [_ w651 w790 w931 w1071 w1211 w1351 w1491 w1631 w1771 w1912]
              tunnel: "YES" -> [_ w650 w789 w930 w1070 w1210 w1350 w1490 w1630 w1770 w1911]
              tunnel: "NO" -> [_ w649 w788 w929 w1069 w1209 w1349 w1489 w1629 w1769 w1910]
              tunnel: w609 -> [_ w646 w787 w927 w1068 w1208 w1348 w1488 w1628 w1768 w1908]
              event Timeout {
                n469 = event-data() -> ()  [unwired: 1 in, 3 out]
              }
              event "RUN LAB01-1": Value Change {
                n470 = event-data() -> ("NewVal"=w647:bool)  [unwired: 1 in, 5 out]
                n471 = local read "SIG LAB01-1"() -> (w648:T2)
                n472 = local write "run lab01-1"(w647) -> ()
                n473 = case shown="True" w647 {
                  tunnel: w657 -> [_ w695]
                  tunnel: w656 -> [_ w694]
                  tunnel: w655 -> [w659 w693]
                  tunnel: w654 -> [_ w692]
                  tunnel: w653 -> [_ w691]
                  tunnel: [w658 w690] -> w652
                  tunnel: w651 -> [_ w689]
                  tunnel: w650 -> [_ w688]
                  tunnel: w649 -> [_ w687]
                  tunnel: w648 -> [_ w686]
                  tunnel: w646 -> [_ w685]
                  frame False {
                    # "stop test"
                    n474 = stacked-sequence {
                      tunnel: w659 -> [_ w671 _]
                      tunnel: [_ w663 _] -> w658
                      frame #0 {
                        n475 = local read "DISP LAB01-1"() -> (w662:T4)
                        n476 = Bundle(cluster=w662, "STATUS"="STOP") -> (w660:T4)  [unwired: 2 in]
                        n477 = local write "DISP LAB01-1"(w660) -> ()
                      }
                      frame #1 {
                        n478 = local read "DISP LAB01-1"() -> (w670:T4)
                        n479 = Unbundle(w670) -> ("CYCLE"=w668:dbl, "MINS"=w669:dbl)  [unwired: 1 out]
                        n480 = case shown="\"CYCLE TEST\"" w671 {
                          tunnel: w669 -> [_ _ w678]
                          tunnel: w668 -> [w676 w677 _]
                          tunnel: [w676 w677 w678] -> w667
                          frame "CHART TEST", Default {
                          }
                          frame "CYCLE TEST" {
                          }
                          frame "T-RISE TEST" {
                          }
                        }
                        n481 = local read "TDMS LAB01-1"() -> (w675:refnum<k34>)
                        n482 = Build Array("STOPPED") -> (w672:string[])
                        n483 = Build Array(w667) -> (w666:dbl[])
                        n484 = TDMS Write(0:w675, 5:"TEST RESULT", 7:w672, 9:w666) -> (4:w664:refnum<k34>, 15:w665:errorcluster)  [unwired: 2 in, 2 out]
                        n485 = TDMS Close(8:w665, 11:w664) -> (0:w663:errorcluster)  [unwired: 1 out]
                      }
                      frame #2 {
                        n486 = stacked-sequence {
                          tunnel: "LAB01-1" -> [w681 w683]
                          frame #0 {
                            n487 = call "sub vi - defrag tdms v1.vi"("panel id"=w681) -> ("error out"=w680:errorcluster)  [unwired: 10 in]
                            n488 = local write "data file error"(w680) -> ()
                          }
                          frame #1 {
                            n489 = call "Save data file (stop) v3.vi"("panel id"=w683) -> ("network file save error"=w682:errorcluster)  [unwired: 9 in, 1 out]
                            n490 = local write "RESULT LAB01-1"(FALSE) -> ()
                            n491 = local write "data file error"(w682) -> ()
                          }
                        }
                      }
                    }
                  }
                  frame True {
                    n492 = stacked-sequence {
                      seq-local: [w697 _] -> [_ w701]
                      tunnel: w695 -> [_ w711]
                      tunnel: w694 -> [_ w710]
                      tunnel: w693 -> [_ w709]
                      tunnel: w692 -> [_ w708]
                      tunnel: w691 -> [_ w707]
                      tunnel: [_ w706] -> w690
                      tunnel: w689 -> [_ w705]
                      tunnel: w688 -> [_ w704]
                      tunnel: w687 -> [_ w703]
                      tunnel: w686 -> [w699 w702]
                      tunnel: w685 -> [_ w700]
                      frame #0 {
                        n493 = Unbundle(w699) -> ("AMPS"=w698:dbl)  [unwired: 4 out]
                        n494 = call "Check For Amps on v1.vi"("ID"="LAB01-1", "amps"=w698) -> ("amps"=w697:bool)  [unwired: 9 in]
                      }
                      frame #1 {
                        n495 = case shown="True" w701 {
                          tunnel: w711 -> [_ w724]
                          tunnel: w710 -> [_ w723]
                          tunnel: w709 -> [_ w722]
                          tunnel: w708 -> [_ w721]
                          tunnel: w707 -> [_ w720]
                          tunnel: [errorcluster {"status"=FALSE, "code"=0, "source"=""} ("error out") w719] -> w706
                          tunnel: w705 -> [_ w718]
                          tunnel: w704 -> [_ w717]
                          tunnel: w703 -> [_ w716]
                          tunnel: w702 -> [_ w715]
                          tunnel: w700 -> [_ w714]
                          frame False {
                            w712 = FALSE
                            n496 = local write "RUN LAB01-1"(w712) -> ()
                            n497 = local write "run lab01-1"(w712) -> ()
                          }
                          frame True {
                            n498 = stacked-sequence {
                              seq-local: [w725 _ _ _ _] -> [_ w746 _ _ _]
                              tunnel: w724 -> [w730 _ _ _ _]
                              tunnel: w723 -> [w726 _ _ _ _]
                              tunnel: w722 -> [w740 _ _ _ _]
                              tunnel: w721 -> [w733 _ _ _ _]
                              tunnel: w720 -> [w728 _ _ _ _]
                              tunnel: [_ w747 _ _ _] -> w719
                              tunnel: w718 -> [_ _ _ w768 _]
                              tunnel: w717 -> [_ _ _ w778 _]
                              tunnel: w716 -> [_ _ _ w777 _]
                              tunnel: w715 -> [_ _ _ _ _]
                              tunnel: w714 -> [_ _ _ _ w784]
                              frame #0 {
                                w727 = "\\"
                                n499 = case shown="\"CHART TEST\", Default" w740 {
                                tunnel: ["L01-1-CHART TEST-" "L01-1-CYCLE TEST-" "L01-1-T-RISE TEST-"] -> w736
                                frame "CHART TEST", Default {
                                }
                                frame "CYCLE TEST" {
                                }
                                frame "T-RISE TEST" {
                                }
                                }
                                n500 = local read "SET LAB01-1"() -> (w735:T5)
                                n501 = Unbundle(w735) -> ("DESCRIPTION"=w734:string)  [unwired: 4 out]
                                n502 = Concatenate Strings(w730, "\\", w728, w727, w726, w727) -> (w737:string)
                                n503 = String To Path(string=w737) -> (path=w739:path)
                                n504 = Concatenate Strings(w737, w736, w734, "-", w733, ".tdms") -> (w725:string)
                                n505 = Create Folder(path (use dialog)=w739) -> (error out=w738:errorcluster)  [unwired: 2 in, 2 out]
                                n506 = call <vilib>:"Clear Errors.vi"("error in (no error)"=w738) -> ()  [unwired: 6 in, 1 out]
                                n507 = global write "Global 1.vi" "LAB01-1 FILE"(w725) -> ()
                              }
                              frame #1 {
                                (unwired) FALSE
                                n508 = String To Path(string=w746) -> (path=w744:path)
                                n509 = TDMS Open(6:FALSE, 10:T20."create or replace" ("operation (0:open)"), 11:w744) -> (0:w747:errorcluster, 3:→"TDMS LAB01-1":refnum<k34>)  [unwired: 4 in]
                              }
                              frame #2 {
                                n510 = local read "TDMS LAB01-1"() -> (w766:refnum<k34>)
                                n511 = local read "SET LAB01-1"() -> (w755:T5)
                                n512 = Build Array("Testers Name", "Description", "Set Test Cycles", "T-Rise minutes", "T-Rise Deg C") -> (w756:string[])
                                n513 = Unbundle(w755) -> ("NAME"=w754:string, "DESCRIPTION"=w753:string, "CYCLES"=w752:dbl, "T-RISE mins"=w751:dbl, "T-RISE deg C"=w750:dbl)
                                n514 = Number To Decimal String(number=w752) -> (decimal integer string=w765:string)  [unwired: 1 in]
                                n515 = Number To Decimal String(number=w751) -> (decimal integer string=w764:string)  [unwired: 1 in]
                                n516 = Number To Decimal String(number=w750) -> (decimal integer string=w763:string)  [unwired: 1 in]
                                n517 = Build Array(w754, w753, w765, w764, w763) -> (w762:string[])
                                n518 = TDMS Set Properties(5:w762, 7:w756, 11:w766) -> ()  [unwired: 3 in, 4 out]
                              }
                              frame #3 {
                                n519 = local read "DISP LAB01-1"() -> (w776:T4)
                                n520 = Concatenate Strings("LAB01-1  ", w768) -> (w767:string)
                                n521 = Two Button Dialog(message=w767, 1:w777, 2:w778) -> (T button?=w770:bool)
                                n522 = case shown="True" w770 {
                                tunnel: w776 -> [w781 w782]
                                tunnel: [w781 w782] -> w775
                                tunnel: [w780 w783] -> w774
                                tunnel: [w779 w783] -> w773
                                frame False {
                                n523 = Unbundle(w781) -> ("CYCLE"=w780:dbl, "MINS"=w779:dbl)  [unwired: 1 out]
                                }
                                frame True {
                                w783 = 0.0
                                }
                                }
                                n524 = Bundle(cluster=w775, "CYCLE"=w774, "MINS"=w773, "STATUS"="RUN") -> (w772:T4)
                                n525 = local write "DISP LAB01-1"(w772) -> ()
                              }
                              frame #4 {
                                n526 = local read "TEMP START LAB01-1"() -> (w786:cluster{"TL":dbl, "TN":dbl})
                                n527 = Bundle(cluster=w786, "TL"=w784, "TN"=w784) -> (w785:cluster{"TL":dbl, "TN":dbl})
                                n528 = local write "TEMP START LAB01-1"(w785) -> ()
                              }
                            }
                          }
                        }
                      }
                    }
                  }
                }
              }
              event "RUN LAB01-2": Value Change {
                n529 = event-data() -> ("NewVal"=w791:bool)  [unwired: 1 in, 5 out]
                n530 = local write "run lab01-2"(w791) -> ()
                n531 = case shown="True" w791 {
                  tunnel: w797 -> [_ w835]
                  tunnel: w796 -> [_ w834]
                  tunnel: w794 -> [w799 w833]
                  tunnel: w795 -> [_ w832]
                  tunnel: w793 -> [_ w831]
                  tunnel: [w798 w830] -> w792
                  tunnel: w790 -> [_ w829]
                  tunnel: w789 -> [_ w828]
                  tunnel: w788 -> [_ w827]
                  tunnel: w787 -> [_ w825]
                  frame False {
                    # "stop test"
                    n532 = stacked-sequence {
                      tunnel: w799 -> [w808 _]
                      tunnel: [w800 _] -> w798
                      frame #0 {
                        n533 = local read "DISP LAB01-2"() -> (w807:T4)
                        n534 = Unbundle(w807) -> ("CYCLE"=w805:dbl, "MINS"=w806:dbl)  [unwired: 1 out]
                        n535 = case shown="\"CHART TEST\", Default" w808 {
                          tunnel: w806 -> [_ _ w815]
                          tunnel: w805 -> [w813 w814 _]
                          tunnel: [w813 w814 w815] -> w804
                          frame "CHART TEST", Default {
                          }
                          frame "CYCLE TEST" {
                          }
                          frame "T-RISE TEST" {
                          }
                        }
                        n536 = local read "TDMS LAB01-2"() -> (w812:refnum<k34>)
                        n537 = Build Array("STOPPED") -> (w809:string[])
                        n538 = Build Array(w804) -> (w803:dbl[])
                        n539 = TDMS Write(0:w812, 5:"TEST RESULT", 7:w809, 9:w803) -> (4:w801:refnum<k34>, 15:w802:errorcluster)  [unwired: 2 in, 2 out]
                        n540 = TDMS Close(8:w802, 11:w801) -> (0:w800:errorcluster)  [unwired: 1 out]
                      }
                      frame #1 {
                        n541 = local read "DISP LAB01-2"() -> (w819:T4)
                        n542 = stacked-sequence {
                          tunnel: "LAB01-2" -> [w821 w823]
                          frame #0 {
                            n543 = call "sub vi - defrag tdms v1.vi"("panel id"=w821) -> ("error out"=w820:errorcluster)  [unwired: 10 in]
                            n544 = local write "data file error"(w820) -> ()
                          }
                          frame #1 {
                            n545 = call "Save data file (stop) v3.vi"("panel id"=w823) -> ("network file save error"=w822:errorcluster)  [unwired: 9 in, 1 out]
                            n546 = local write "RESULT LAB01-2"(FALSE) -> ()
                            n547 = local write "data file error"(w822) -> ()
                          }
                        }
                        n548 = Bundle(cluster=w819, "STATUS"="STOP") -> (w817:T4)  [unwired: 2 in]
                        n549 = local write "DISP LAB01-2"(w817) -> ()
                      }
                    }
                  }
                  frame True {
                    n550 = local read "SIG LAB01-2"() -> (w826:T2)
                    n551 = stacked-sequence {
                      seq-local: [w837 _] -> [_ w841]
                      tunnel: w835 -> [_ w851]
                      tunnel: w834 -> [_ w850]
                      tunnel: w833 -> [_ w849]
                      tunnel: w832 -> [_ w848]
                      tunnel: w831 -> [_ w847]
                      tunnel: [_ w846] -> w830
                      tunnel: w829 -> [_ w845]
                      tunnel: w828 -> [_ w844]
                      tunnel: w827 -> [_ w843]
                      tunnel: w826 -> [w836 w842]
                      tunnel: w825 -> [_ w840]
                      frame #0 {
                        n552 = Unbundle(w836) -> ("AMPS"=w839:dbl)  [unwired: 4 out]
                        n553 = call "Check For Amps on v1.vi"("ID"="LAB01-2", "amps"=w839) -> ("amps"=w837:bool)  [unwired: 9 in]
                      }
                      frame #1 {
                        n554 = case shown="True" w841 {
                          tunnel: w851 -> [_ w864]
                          tunnel: w850 -> [_ w863]
                          tunnel: w849 -> [_ w862]
                          tunnel: w848 -> [_ w861]
                          tunnel: w847 -> [_ w860]
                          tunnel: [errorcluster {"status"=FALSE, "code"=0, "source"=""} ("error out") w859] -> w846
                          tunnel: w845 -> [_ w858]
                          tunnel: w844 -> [_ w857]
                          tunnel: w843 -> [_ w856]
                          tunnel: w842 -> [_ w855]
                          tunnel: w840 -> [_ w854]
                          frame False {
                            w852 = FALSE
                            n555 = local write "RUN LAB01-2"(w852) -> ()
                            n556 = local write "run lab01-2"(w852) -> ()
                          }
                          frame True {
                            n557 = stacked-sequence {
                              seq-local: [w865 _ _ _ _] -> [_ w889 _ _ _]
                              tunnel: w864 -> [w870 _ _ _ _]
                              tunnel: w863 -> [w867 _ _ _ _]
                              tunnel: w862 -> [w880 _ _ _ _]
                              tunnel: w861 -> [w873 _ _ _ _]
                              tunnel: w860 -> [w868 _ _ _ _]
                              tunnel: [_ w884 _ _ _] -> w859
                              tunnel: w858 -> [_ _ _ w911 _]
                              tunnel: w857 -> [_ _ _ w910 _]
                              tunnel: w856 -> [_ _ _ w909 _]
                              tunnel: w855 -> [_ _ _ _ _]
                              tunnel: w854 -> [_ _ _ _ w924]
                              frame #0 {
                                w866 = "\\"
                                n558 = local read "SET LAB01-2"() -> (w875:T5)
                                n559 = case shown="\"CYCLE TEST\"" w880 {
                                tunnel: ["L01-2-CHART TEST-" "L01-2-CYCLE TEST-" "L01-2-T-RISE TEST-"] -> w876
                                frame "CHART TEST", Default {
                                }
                                frame "CYCLE TEST" {
                                }
                                frame "T-RISE TEST" {
                                }
                                }
                                n560 = Unbundle(w875) -> ("DESCRIPTION"=w874:string)  [unwired: 4 out]
                                n561 = Concatenate Strings(w870, "\\", w868, w866, w867, w866) -> (w877:string)
                                n562 = String To Path(string=w877) -> (path=w879:path)
                                n563 = Concatenate Strings(w877, w876, w874, "-", w873, ".tdms") -> (w865:string)
                                n564 = Create Folder(path (use dialog)=w879) -> (error out=w878:errorcluster)  [unwired: 2 in, 2 out]
                                n565 = call <vilib>:"Clear Errors.vi"("error in (no error)"=w878) -> ()  [unwired: 6 in, 1 out]
                                n566 = global write "Global 1.vi" "LAB01-2 FILE"(w865) -> ()
                              }
                              frame #1 {
